vi "FIR_2decimate_125cycles.vi"(7 "reset":bool, 8 "valid in":bool, 10 "Q in":fxp<+/-,16,14>, 11 "I in":fxp<+/-,16,14>) -> (0 "valid out":bool, 2 "Q out":fxp<+/-,16,14>, 3 "I out":fxp<+/-,16,14>, 4 "ready for input":bool)   [LabVIEW 2013]
uses:
  <vilib>/rvi/FXPMathLib/FxpConvert/subVIs/nifxpmath_Convert_SimConfig.ctl
  <vilib>/fxp/LVFixedPointQuantizationPolicyTypeDef.ctl
  <vilib>/fxp/LVFixedPointOverflowPolicyTypeDef.ctl
  <vilib>/rvi/IPIntegrationNode/IPINode_Utilities/niFpgaIPINodeSimCore.vi
  <vilib>/rvi/FXPMathLib/FxpConvert/simVIs/DllFxpConvertTemp_sub.vi
  <vilib>/rvi/XilinxIP/XIPIN_XNode/niFpgaXIPIN.xnode
  Filters/FIR_2decimate_125cycles/FIR_2decimate_125cycles_A5F5B967F2844EBF91F2B7F364D8D5CB.dll
  <vilib>/rvi/IPIntegrationNode/IPINode_Xnode/niFpgaIPINode.xnode
  <vilib>/rvi/FXPMathLib/FxpInterpret/XNode/nifxpmath_Interpret.xnode
  <vilib>/rvi/FXPMathLib/FxpConvert/XNode/nifxpmath_Convert.xnode
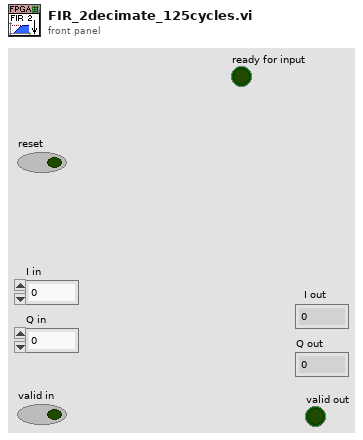
[diagram p1: front panel]
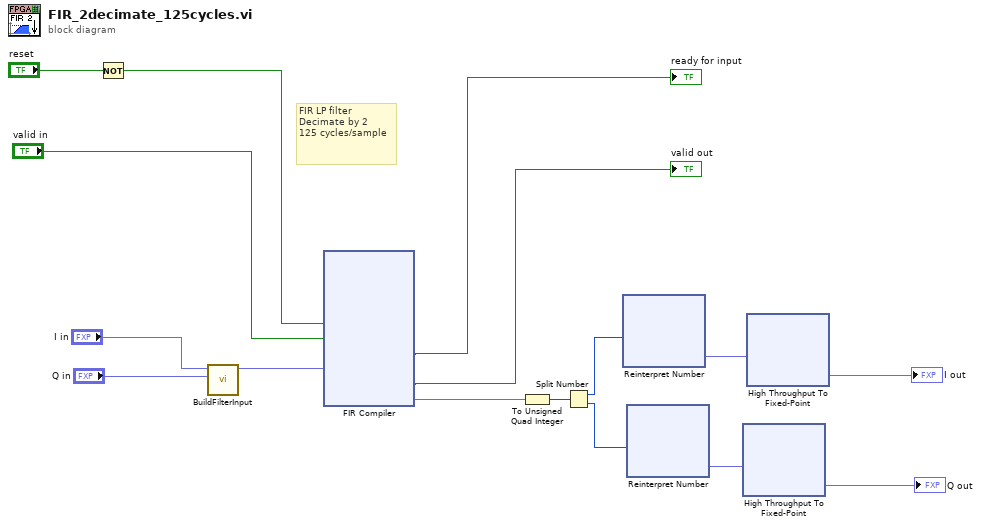
[diagram p0: block diagram]
diagram:
  # "FIR LP filter\nDecimate by 2\n125 cycles/sample"
  n1 = Not(x="reset") -> (.not. x?=w13:bool)
  n2 = call "BuildFilterInput.vi"("Q in"="Q in", "I in"="I in") -> ("Filter input"=w11:fxp<+,32,32>)  [unwired: 9 in]
  n3 = xnode ("FIR Compiler")("aresetn"=w13, "s_axis_data_tvalid"="valid in", "s_axis_data_tdata"=w11) -> ("s_axis_data_tready"=→"ready for input":bool, "m_axis_data_tvalid"=→"valid out":bool, "m_axis_data_tdata"=w3:fxp<+,64,64>)  [unwired: 1 in]
  n4 = To Unsigned Quad Integer(1:w3) -> (0:w7:u64)
  n5 = Split Number(x=w7) -> (hi(x)=w8:u32, lo(x)=w4:u32)
  n6 = xnode "Reinterpret Number"("x"=w8) -> ("y"=w5:fxp<+/-,32,16>)
  n7 = xnode "Reinterpret Number"("x"=w4) -> ("y"=w6:fxp<+/-,32,16>)
  n8 = xnode "High Throughput To Fixed-Point"("x"=w6) -> ("y"=→"Q out":fxp<+/-,16,14>)
  n9 = xnode "High Throughput To Fixed-Point"("x"=w5) -> ("y"=→"I out":fxp<+/-,16,14>)
